vi "Read Encoders 2.vi"(8 "error in (no error)":errorcluster, 9 "No samples":u32=1000, 11 "task in":i32) -> (0 "error out":errorcluster, 1 "CW/CCW":bool, 2 "Not rotating":bool, 3 "task out":i32)   [LabVIEW 2023]
uses:
  <userlib>/DAQNavi Polymorphic VI/read/DAQNavi Read (Digital 1D Wfm NChan NSamp).vi
panel:
  in  "DUT1":bool
  out "data":digitalwaveform[](array[waveform])
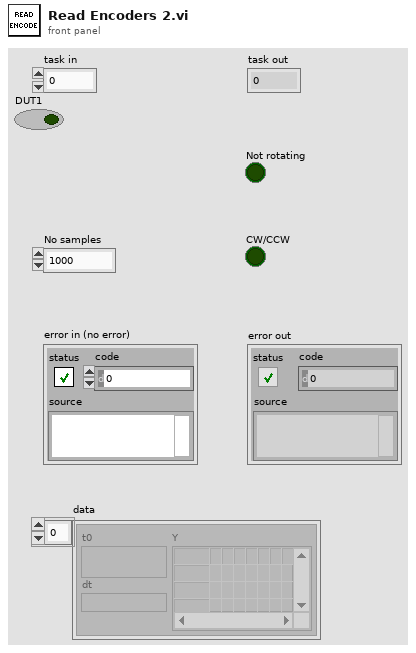
[diagram p1: front panel]
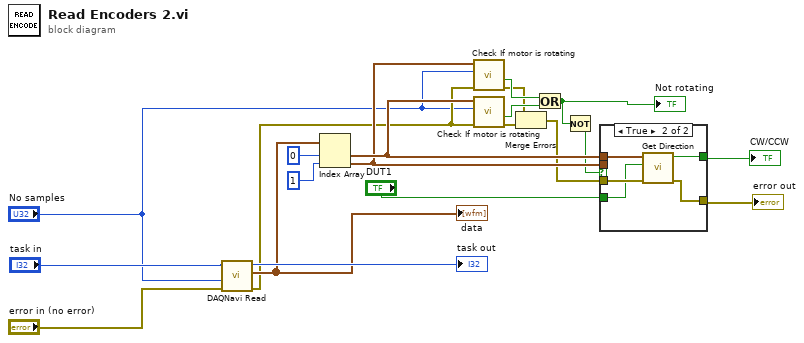
[diagram p0: block diagram]
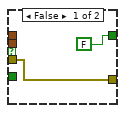
[diagram p2: hidden frame]
diagram:
  n1 = call-poly <userlib>:"DAQNavi Read.vi"("error in (no error)"="error in (no error)", "number of samples per channel to read"="No samples", "task in"="task in") -> ("error out"=w9:errorcluster, "data"=w17:digitalwaveform[], "task out"=→"task out":i32)  [unwired: 1 in, 5 out]
  "data" <- w17
  n2 = Index Array(array=w17, index #1=0 ("index"), index #2=1 ("index")) -> (element #1=w13:digitalwaveform, element #2=w10:digitalwaveform)
  n3 = call "Check If motor is rotating.vi"("error in (no error)"=w9, "No samples"="No samples", "Encoder signal"=w10) -> ("error out"=w4:errorcluster, "Not rotating"=w6:bool)  [unwired: 6 in, 1 out]
  n4 = call "Check If motor is rotating.vi"("error in (no error)"=w9, "No samples"="No samples", "Encoder signal"=w13) -> ("error out"=w12:errorcluster, "Not rotating"=w7:bool)  [unwired: 6 in, 1 out]
  n5 = Merge Errors(w4, w12) -> (w5:errorcluster)
  n6 = Or(x=w6, y=w7) -> (x .or. y?=w3:bool)
  "Not rotating" <- w3
  n7 = Not(x=w3) -> (.not. x?=w2:bool)
  n8 = case shown="True" w2 {
    tunnel: [FALSE ("CW/CCW") w27] -> w14
    tunnel: w13 -> [_ w26]
    tunnel: [w21 w25] -> w11
    tunnel: w10 -> [_ _]
    tunnel: w5 -> [w21 w24]
    tunnel: "DUT1" -> [_ w23]
    frame False {
    }
    frame True {
      n9 = call "Get Direction.vi"("error in (no error)"=w24, "DUT1"=w23, "Measured signal"=w26) -> ("error out"=w25:errorcluster, "CW/CCW"=w27:bool)  [unwired: 6 in, 1 out]
    }
  }
  "error out" <- w11
  "CW/CCW" <- w14
